vi "Update Plugin Status.vi"(8 "error in (no error)":errorcluster, 11 "CIF_UI in":refnum<class "CIF_UI.lvclass">) -> (0 "error out":errorcluster, 3 "CIF_UI out":refnum<class "CIF_UI.lvclass">)   [LabVIEW 2021, in "CIF_UI.lvclass"]
uses:
  CIF_UI.lvclass
  CIF_UI.lvclass/CIF_UI.ctl
  <vilib>/Utility/miscctls.llb/LVMapReplaceAction.ctl
  CIFPluginManager/CIFPluginManager/gRPC/CIF_Manager_Client_Wrapper/CIFManagerClientWrapper.lvlib
  CIFCore/Grpc/CIFCoreWrapper/CIFCoreWrapper.lvlib
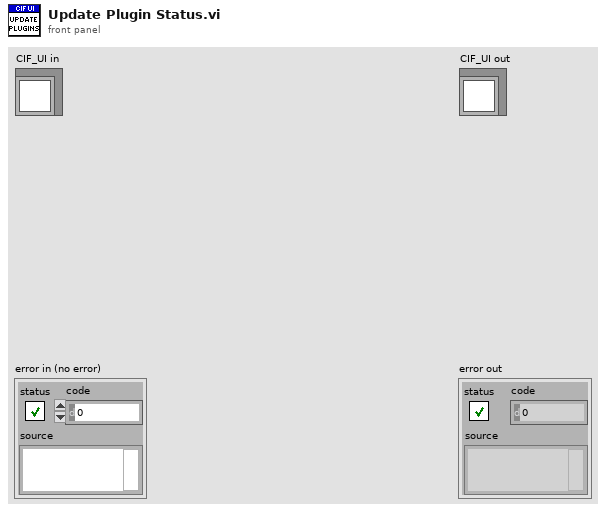
[diagram p1: front panel]
types:
  T1 = typedef "LVMapReplaceAction.ctl" = enum32{"Modify Entry only if found", "Add or Modify Entry", "Delete Entry"}
  T2 = typedef "grpc-lvsupport-release.lvlib/grpcId.ctl" = u64
  T3 = typedef "CIF_UI.lvclass/Plugin Connection Map.ctl" = map{string, T4}
  T4 = typedef "CIF_UI.lvclass/Plugin Connections.ctl" = cluster{"gRPC ID":T2, "Plugin info":T5}
  T5 = typedef "CIF_Manager_client.lvlib/cif_manager_PluginInfo.ctl" = cluster{"plugin_name":string, "plugin_type":string, "grpc_port":i32, "plugin_version":T6, "status":T7}
  T6 = typedef "CIF_Manager_client.lvlib/cif_manager_PluginVersion.ctl" = cluster{"major_version":i32, "minor_version":i32, "fix_version":i32, "build_version":i32}
  T7 = typedef "CIF_Manager_client.lvlib/cif_plugincore_StatusData.ctl" = cluster{"state":T8, "timing_statistics":T9, "fifo_statistics":T11, "error":T12, "monitor_doubles":T13, "monitor_u64s":T14, "monitor_i64s":T15}
  T8 = typedef "CIF_Manager_client.lvlib/cif_plugincore_StatusData_State.ctl" = enum32{"NULL", "CREATING", "LISTENING", "RUNNING", "CLEANINGUP", "DESTROYING"}
  T9 = typedef "CIF_Manager_client.lvlib/cif_plugincore_TimingStatistics.ctl" = cluster{"period":T10, "wake_error":T10, "execute":T10, "housekeep":T10, "idle":T10}
  T10 = typedef "CIF_Manager_client.lvlib/cif_plugincore_TimingStatsBasic.ctl" = cluster{"max":i32, "min":i32}
  T11 = typedef "CIF_Manager_client.lvlib/cif_plugincore_FifoStatistics.ctl" = cluster{"from_t0":T10, "from_previous_plugin":T10, "output_error":T10}
  T12 = typedef "CIF_Manager_client.lvlib/cif_plugincore_Error.ctl" = cluster{"status":bool, "code":i32}
  T13 = typedef "CIF_Manager_client.lvlib/cif_plugincore_MonitorDoubles.ctl" = cluster{"double_1":dbl, "double_2":dbl, "double_3":dbl, "double_4":dbl}
  T14 = typedef "CIF_Manager_client.lvlib/cif_plugincore_MonitorU64.ctl" = cluster{"u64_1":u64, "u64_2":u64, "u64_3":u64, "u64_4":u64}
  T15 = typedef "CIF_Manager_client.lvlib/cif_plugincore_MonitorI64.ctl" = cluster{"i64_1":i64, "i64_2":i64, "i64_3":i64, "i64_4":i64}
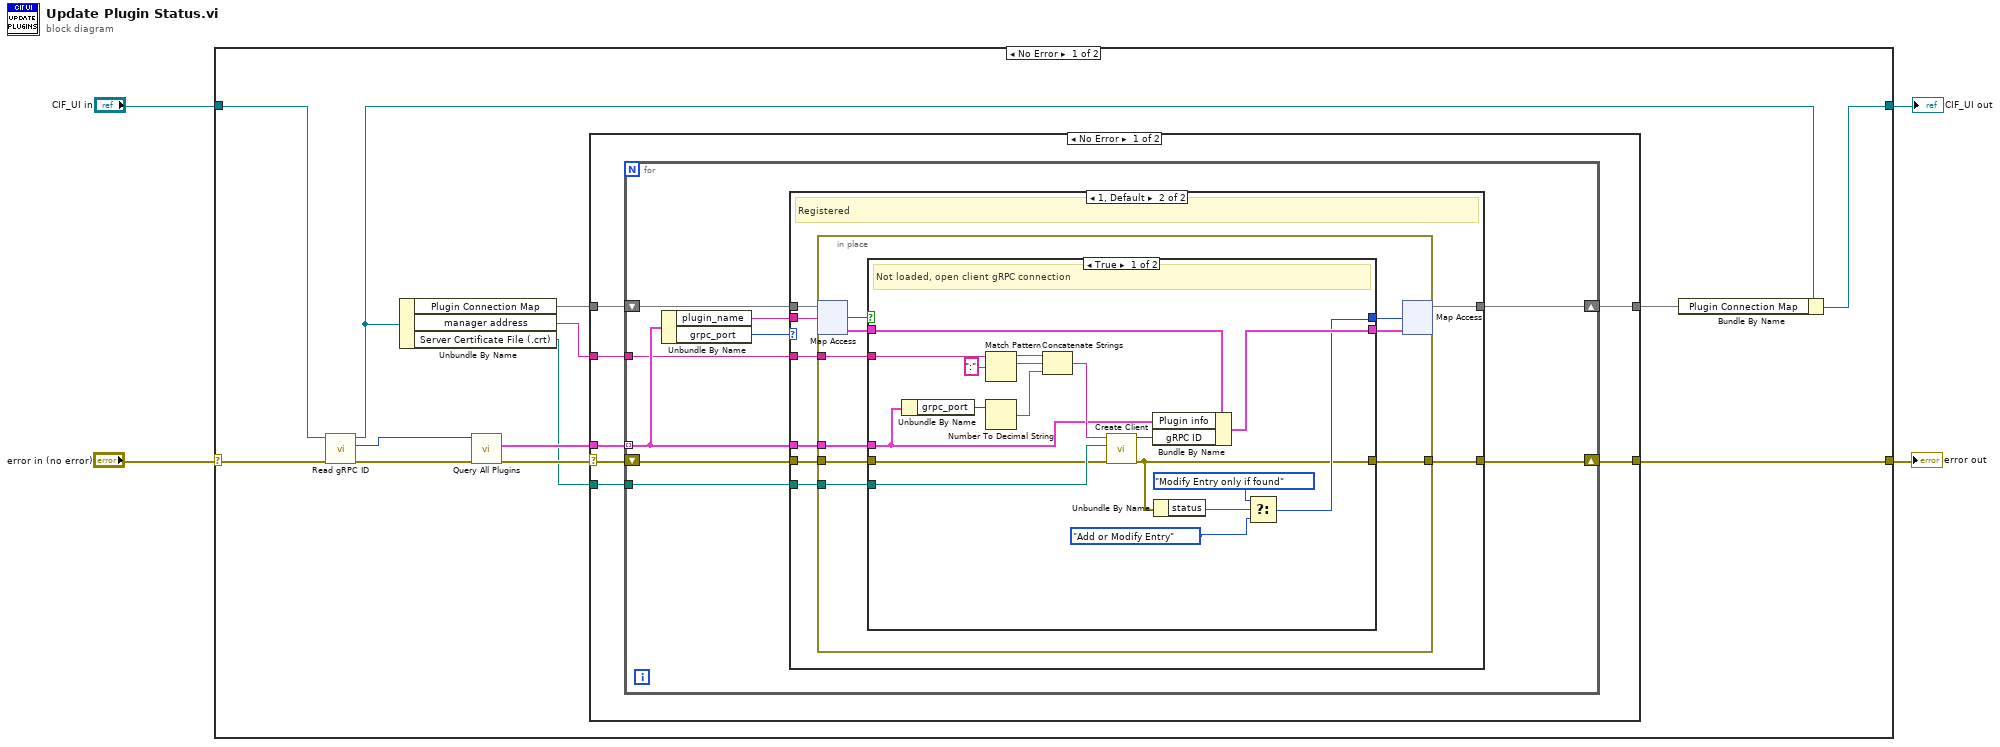
[diagram p0: block diagram]
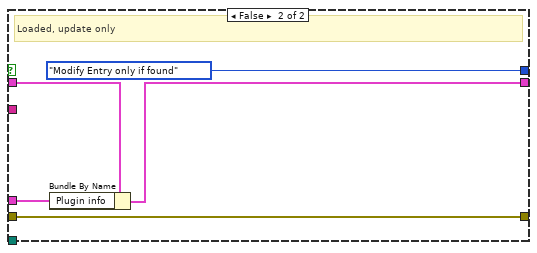
[diagram p3: hidden frame]
diagram:
  n1 = case shown="No Error" "error in (no error)" {
    selector: "error in (no error)" -> [w14 w79]
    tunnel: [w8 w79] -> w3
    tunnel: [w5 w78] -> w1
    tunnel: "CIF_UI in" -> [w15 w78]
    frame No Error {
      n2 = call "Read gRPC ID.vi"("error in (no error)"=w14, "CIF_UI in"=w15) -> ("error out"=w16:errorcluster, "gRPCid"=w17:T2, "CIF_UI out"=w7:refnum<class "CIF_UI.lvclass">)  [unwired: 7 in]
      n3 = Unbundle By Name(w7) -> ("Plugin Connection Map"=w11:T3, "manager address"=w10:string, "Server Certificate File (.crt)"=w9:path)
      n4 = call "Query All Plugins.vi"("error in"=w16, "gRPC ID in"=w17) -> ("error out"=w13:errorcluster, "plugin_info"=w12:T5[])  [unwired: 7 in, 1 out]
      n5 = case shown="No Error" w13 {
        selector: w13 -> [w20 w77]
        tunnel: w12 -> [w24 _]
        tunnel: w11 -> [w23 w76]
        tunnel: w10 -> [w22 _]
        tunnel: w9 -> [w21 _]
        tunnel: [w19 w77] -> w8
        tunnel: [w18 w76] -> w6
        frame No Error {
          n6 = for {
            tunnel: w24 -> [w31] mode=indexing
            tunnel: w22 -> [w30]
            tunnel: w21 -> [w29]
            shift-right: [w26] -> w19
            shift-left: w20 -> [w28]
            shift-right: [w25] -> w18
            shift-left: w23 -> [w33]
            n7 = Unbundle By Name(w31) -> ("plugin_name"=w32:string, "grpc_port"=w27:i32)
            n8 = case shown="1, Default" w27 {
              tunnel: w33 -> [w35 w43]
              tunnel: w32 -> [_ w42]
              tunnel: w31 -> [_ w41]
              tunnel: w30 -> [_ w40]
              tunnel: w29 -> [_ w39]
              tunnel: w28 -> [w34 w38]
              tunnel: [w34 w37] -> w26
              tunnel: [w35 w36] -> w25
              frame -1, 0 {
                # "Not a valid port.  Not yet registered"
              }
              frame 1, Default {
                # "Registered"
                n9 = in-place {
                  in-place-border: w41 -> [w51]
                  in-place-border: w40 -> [w49]
                  in-place-border: w39 -> [w48]
                  in-place-border: w38 -> [w47]
                  in-place-border: [w44] -> w37
                  n10 = in-place-map #1(w43, w42) -> (w50:T4, w52:bool)  [unwired: 1 in]
                  n11 = case shown="True" w52 {
                    tunnel: w51 -> [w60 w74]
                    tunnel: w50 -> [w61 w75]
                    tunnel: w49 -> [w69 _]
                    tunnel: w48 -> [w63 _]
                    tunnel: w47 -> [w62 w71]
                    tunnel: [w58 w73] -> w46
                    tunnel: [w54 LVMapReplaceAction."Modify Entry only if found" ("action")] -> w45
                    tunnel: [w53 w71] -> w44
                    frame True {
                      # "Not loaded, open client gRPC connection"
                      n12 = Unbundle By Name(w60) -> ("grpc_port"=w70:i32)
                      n13 = Match Pattern(string=w69, regular expression=":") -> (before substring=w67:string, match substring=w65:string)  [unwired: 1 in, 2 out]
                      n14 = Number To Decimal String(number=w70) -> (decimal integer string=w66:string)  [unwired: 1 in]
                      n15 = Concatenate Strings(w67, w65, w66) -> (w64:string)
                      n16 = call "Create Client.vi"("error in"=w62, "Server Certificate File (.crt)"=w63, "address"=w64) -> ("error out"=w53:errorcluster, "gRPC ID Out"=w59:T2)  [unwired: 7 in]
                      n17 = Bundle By Name(cluster=w61, "Plugin info"=w60, "gRPC ID"=w59) -> (w58:T4)
                      n18 = Unbundle By Name(w53) -> ("status"=w57:bool)
                      n19 = Select(t=LVMapReplaceAction."Modify Entry only if found", s=w57, f=LVMapReplaceAction."Add or Modify Entry" ("action")) -> (s? t:f=w54:T1)
                    }
                    frame False {
                      # "Loaded, update only"
                      n20 = Bundle By Name(cluster=w75, "Plugin info"=w74) -> (w73:T4)
                    }
                  }
                  n21 = in-place-map #1(w46, w45) -> (w36:T3)  [unwired: 2 out]
                }
              }
            }
          }
        }
        frame Error {
        }
      }
      n22 = Bundle By Name(cluster=w7, "Plugin Connection Map"=w6) -> (w5:refnum<class "CIF_UI.lvclass">)
    }
    frame Error {
    }
  }
  "error out" <- w3
  "CIF_UI out" <- w1
